vi "Magnetic Sweep 1.5.vi"() -> ()   [LabVIEW 2011]
uses:
  <vilib>/Math Plots/3D Math Plots/3D Contour/3D Contour XCtrl/3D Contour.xctl
  <vilib>/Math Plots/3D Math Plots/3D Contour/3D Contour Datatype/Public/Plot Helper (Vector).vi
  <vilib>/Math Plots/3D Math Plots/3D Contour/3D Contour Datatype/3D Contour Datatype.lvclass
panel:
  out "Heater":bool
  out "Persistent switch ready":bool
  out "error out 6":errorcluster
  in  "Temperature\nlower limite":dbl
  out "Ramping rate command":string
  out "Target field command":string
  out "error out 5":errorcluster
  in  "error out 4":errorcluster
  out "String":string="Persistent switch is not on"
  in  "Set parameter":bool
  out "status":string
  out "PID command":string
  out "setpoint command":string
  out "setpoint":dbl
  out "3D Contour \n(Ramp down)":refnum<class "3D Plot Datatype.lvclass">[](xcontrol)
  out "3D Contour\n(Ramp up)":refnum<class "3D Plot Datatype.lvclass">[](xcontrol)
  in  "stop":bool
  out "error out 3":errorcluster
  out "error out 2":errorcluster
  in  "Contour plot (ramp down)":path
  in  "Raw data (ramp down)":path
  out "Elapsed Time (s)":dbl
  out "Iteration":i32
  in  "error out":errorcluster
  out "Initial Temperature":string
  out "Zero field reached":bool
  out "Target field reached":bool
  in  "Temperature\nupper limite":dbl
  in  "Temperature\nramping step":dbl
  in  "Heater range":i16(ring) items=["High", "Medium", "Low"]
  in  "D gain":dbl
  in  "I gain":dbl
  in  "P gain":dbl
  in  "Contour plot (ramp up)":path
  out "Time elapsed":string
  in  "Timer":bool caption="Reset"
  in  "date format":enum16{"short", "long", "abbreviated"}(ring)
  in  "Save":bool
  in  "Raw data (ramp  up)":path
  out "Temperature vs Time":cluster{dbl[], dbl[]}(graph)
  out "current time":timestamp
  out "Magnetic\nField":cluster{dbl[], dbl[]}(graph)
  out "Current Resistance":string
  out "Current Temperature":string
  out "Current Field":string
  out "Status":string
  in  "Field Sweep":bool
  in  "Magnetic field\nRamp rate":dbl
  in  "Traget Field":dbl
  out "Init Response":string
  in  "error in (no error)":errorcluster
  in  "IP Address":string
  in  "Ramp":bool
  in  "Update":bool
  in  "Ramp to Zero":bool
  in  "P Switch":bool
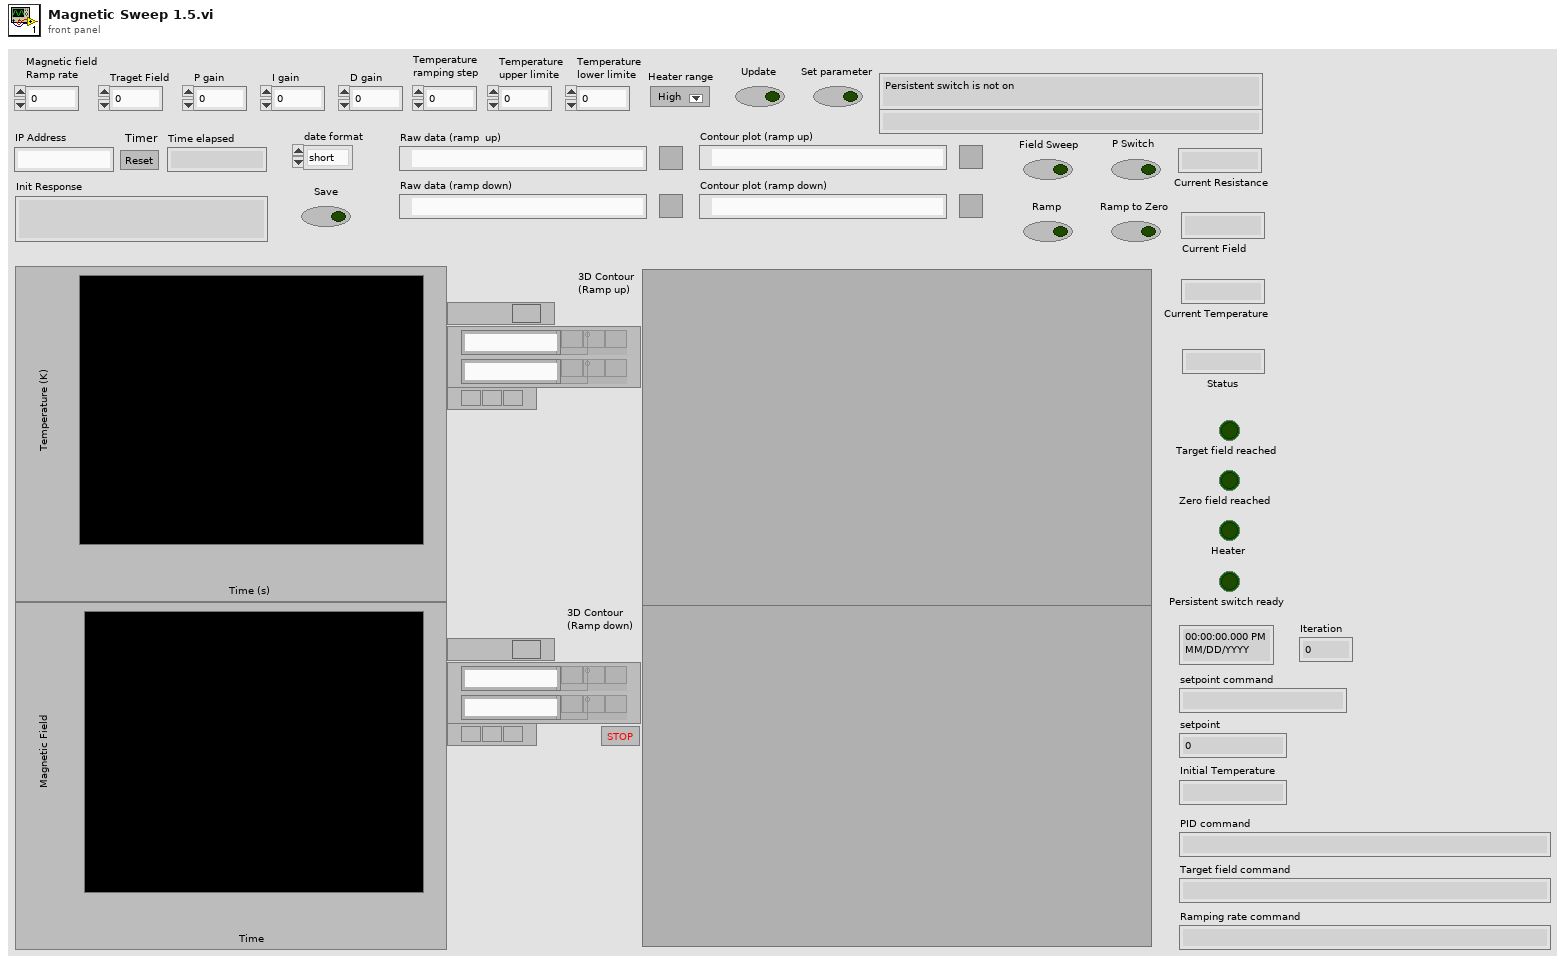
[diagram p1: front panel]
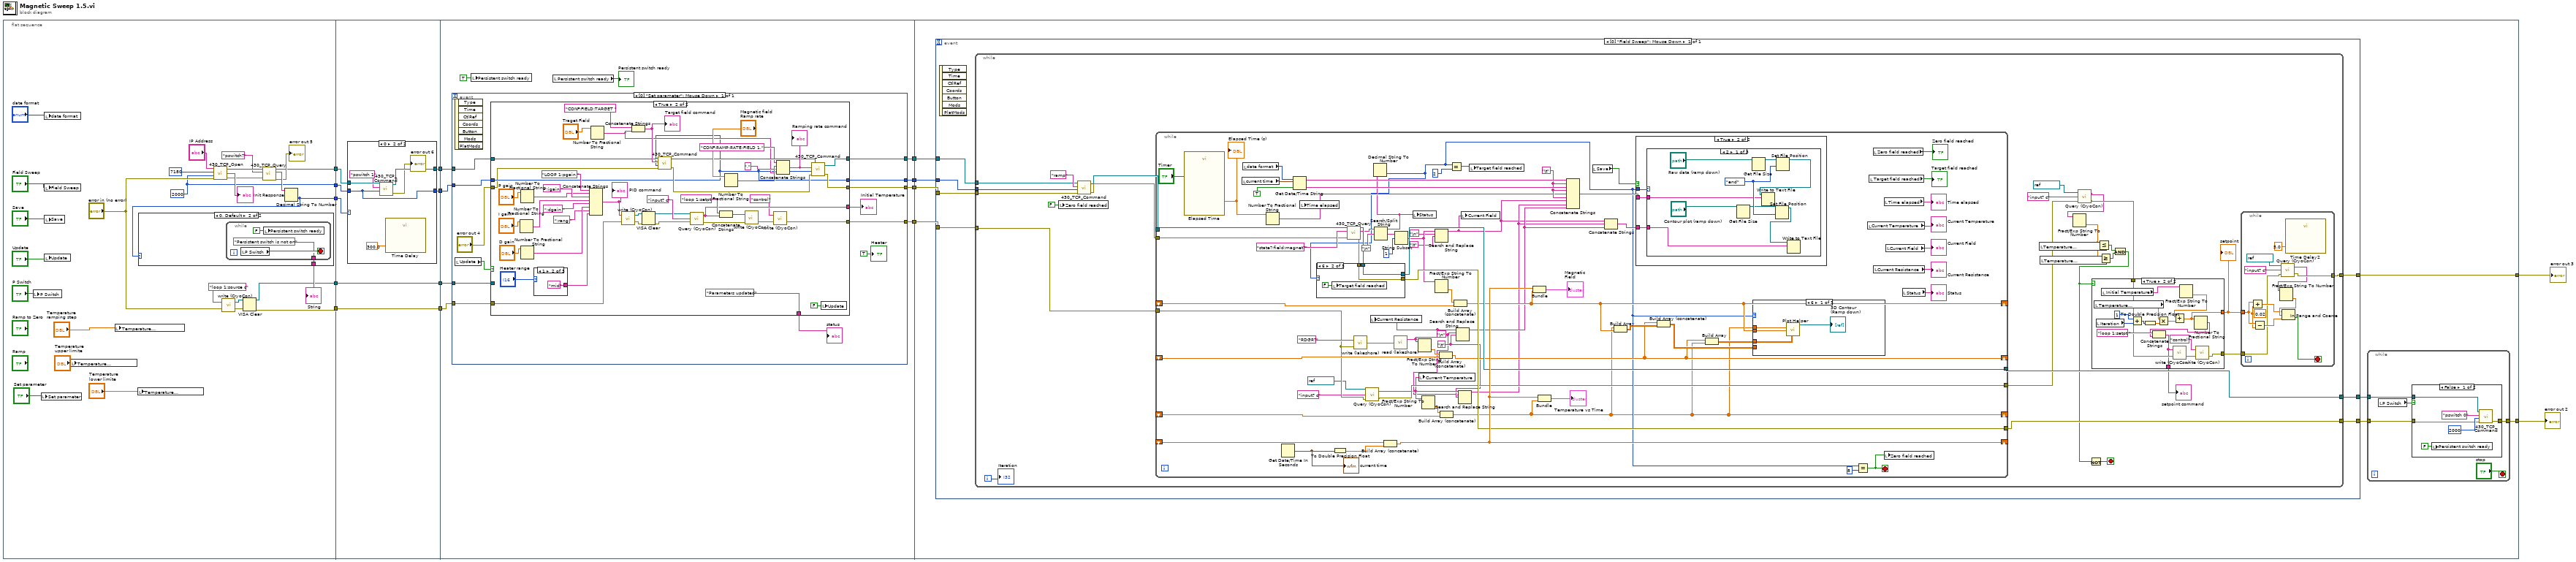
[diagram p0: block diagram]
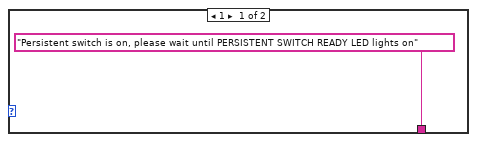
[diagram p2: hidden frame]
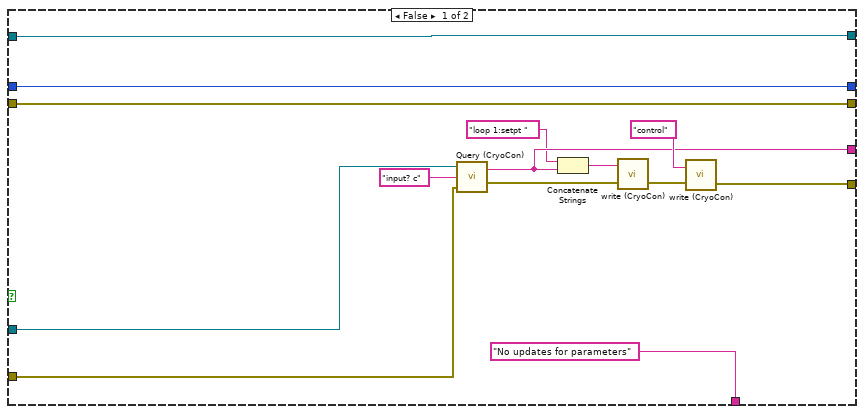
[diagram p4: hidden frame]
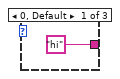
[diagram p5: hidden frame]
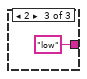
[diagram p6: hidden frame]
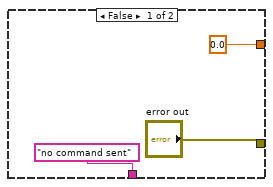
[diagram p8: hidden frame]
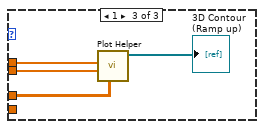
[diagram p10: hidden frame]
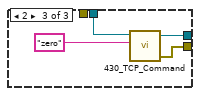
[diagram p12: hidden frame]
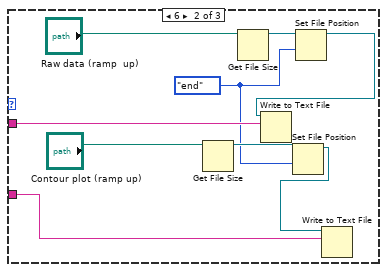
[diagram p14: hidden frame]
diagram:
  n1 = flat-sequence {
    tunnel: [w17] -> w9
    tunnel: [w20] -> w7
    tunnel: [w23] -> w5
    tunnel: [w21] -> w3
    tunnel: [w16] -> w1
    tunnel: w9 -> [w52]
    tunnel: [w50] -> w8
    tunnel: w7 -> [w51]
    tunnel: [w48] -> w6
    tunnel: w5 -> [w54]
    tunnel: [w54] -> w4
    tunnel: w3 -> [w53]
    tunnel: [w53] -> w2
    tunnel: w1 -> [w49]
    tunnel: w8 -> [w72]
    tunnel: w6 -> [w71]
    tunnel: w4 -> [w70]
    tunnel: [w69] -> w15
    tunnel: [w68] -> w12
    tunnel: [w67] -> w11
    tunnel: [w66] -> w10
    tunnel: w2 -> [w65]
    tunnel: w15 -> [w154]
    tunnel: [w153] -> w14
    tunnel: [w151] -> w13
    tunnel: w12 -> [w149]
    tunnel: w11 -> [w148]
    tunnel: w10 -> [w147]
    frame #0 {
      w20 = 2000 ("Timeout")
      n2 = local write "P Switch"("P Switch") -> ()
      n3 = local write "Set parameter"("Set parameter") -> ()
      n4 = local write "date format"("date format") -> ()
      n5 = local write "Field Sweep"("Field Sweep") -> ()
      n6 = local write "Save"("Save") -> ()
      n7 = local write "Update"("Update") -> ()
      n8 = local write "Temperature\nupper limite"("Temperature\nupper limite") -> ()
      n9 = local write "Temperature\nramping step"("Temperature\nramping step") -> ()
      n10 = local write "Temperature\nlower limite"("Temperature\nlower limite") -> ()
      n11 = call "430_TCP_Open.vi"("IP Address"="IP Address", "TCP Port"=7180, "timeout ms (2000)"=w20, "error in (no error)"="error in (no error)") -> ("connection ID"=w30:refnum<k5>, "Init Response"=→"Init Response":string, "error out"=w29:errorcluster)  [unwired: 2 in]
      n12 = call "write (CryoCon).vi"("error in (no error)"="error in (no error)", "write buffer"="loop 1:source c") -> ("error out"=w25:errorcluster, "VISA resource name out"=w24:refnum<visa-resource-name>)
      n13 = VISA Clear(VISA resource name=w24, error in (no error)=w25) -> (VISA resource name out=w21:refnum<visa-resource-name>, error out=w23:errorcluster)
      n14 = call "430_TCP_Query.vi"("error in (no error)"=w29, "Command"="pswitch?", "connection ID"=w30) -> ("error out"=→"error out 5":errorcluster, "Response"=w27:string, "connection ID out"=w17:refnum<k5>)  [unwired: 4 in, 2 out]
      n15 = Decimal String To Number(string=w27) -> (number=w16:i32)  [unwired: 2 in, 1 out]
      n16 = case shown="0, Default" w16 {
        tunnel: ["Persistent switch is on, please wait until PERSISTENT SWITCH READY LED lights on" w44] -> w22
        frame 1 {
        }
        frame 0, Default {
          n17 = while {
            tunnel: ["Persistent switch is not on"] -> w44
            stop <- w47 stop-if-true
            n18 = local read "P Switch"() -> (w47:bool)
            n19 = local write "Persistent switch ready"(FALSE ("Persistent switch ready")) -> ()
          }
        }
      }
      "String" <- w22
    }
    frame #1 {
      n20 = case shown="0" w49 {
        tunnel: w52 -> [w56 w62]
        tunnel: w51 -> [w55 w57]
        tunnel: [w56 w61] -> w50
        tunnel: [w55 w57] -> w48
        frame 1, Default {
        }
        frame 0 {
          n21 = call "430_TCP_Command.vi"("Timeout"=w57, "Command"="pswitch 1", "connection ID"=w62) -> ("error out"=→"error out 6":errorcluster, "connection ID out"=w61:refnum<k5>)  [unwired: 1 in, 1 out]
          n22 = call "Time Delay"("Delay Time (s)"=300.0) -> ()  [unwired: 10 in, 1 out]
        }
      }
    }
    frame #2 {
      n23 = event shown="[0] \"Set parameter\": Mouse Down" {
        selector: _ -> [_]
        dyn-events: _ -> [_]
        timeout: _ -> [_]
        tunnel: w72 -> [w85]
        tunnel: w71 -> [w84]
        tunnel: w70 -> [w83]
        tunnel: [w82] -> w69
        tunnel: [w81] -> w68
        tunnel: [w80] -> w67
        tunnel: [w79] -> w66
        tunnel: w65 -> [w75]
        event "Set parameter": Mouse Down {
          n24 = event-data() -> ()  [unwired: 1 in, 7 out]
          n25 = local read "Update"() -> (w76:bool)
          n26 = case shown="True" w76 {
            tunnel: w85 -> [w97 w141]
            tunnel: w84 -> [w98 w113]
            tunnel: w83 -> [w94 w120]
            tunnel: [w86 w101] -> w82
            tunnel: ["No updates for parameters" ("String") "Parameters updated" ("String")] -> w78
            tunnel: [w93 w115] -> w81
            tunnel: [w97 w114] -> w80
            tunnel: [w98 w113] -> w79
            tunnel: [w89 w105] -> w77
            tunnel: w75 -> [w95 _]
            tunnel: "error out 4" -> [w93 w100]
            frame False {
              n27 = call "Query (CryoCon).vi"("error in (no error)"=w94, "write buffer"="input? c", "VISA resource name 2"=w95) -> ("error out"=w87:errorcluster, "read buffer"=w89:string)
              n28 = Concatenate Strings("loop 1:setpt " ("write buffer"), w89) -> (w92:string)
              n29 = call "write (CryoCon).vi"("error in (no error)"=w87, "write buffer"=w92) -> ("error out"=w91:errorcluster)  [unwired: 1 out]
              n30 = call "write (CryoCon).vi"("error in (no error)"=w91, "write buffer"="control") -> ("error out"=w86:errorcluster)  [unwired: 1 out]
            }
            frame True {
              n31 = Number To Fractional String(number="I gain") -> (F-format string=w124:string)  [unwired: 3 in]
              n32 = Number To Fractional String(number="D gain") -> (F-format string=w122:string)  [unwired: 3 in]
              n33 = Number To Fractional String(number="P gain") -> (F-format string=w125:string)  [unwired: 3 in]
              n34 = case shown="1" "Heater range" {
                tunnel: ["hi" "mid" "low"] -> w117
                frame 0, Default {
                }
                frame 1 {
                }
                frame 2 {
                }
              }
              n35 = Concatenate Strings("LOOP 1:pgain " ("write buffer"), w125, ";igain " ("string"), w124, ";dgain " ("string"), w122, ";rang " ("string"), w117) -> (w121:string)
              "PID command" <- w121
              n36 = Number To Fractional String(number="Traget Field") -> (F-format string=w131:string)  [unwired: 3 in]
              n37 = call "write (CryoCon).vi"("error in (no error)"=w120, "write buffer"=w121) -> ("error out"=w112:errorcluster, "VISA resource name out"=w111:refnum<visa-resource-name>)
              n38 = Concatenate Strings("CONF:FIELD:TARGET ", w131) -> (w142:string)
              "Target field command" <- w142
              n39 = VISA Clear(VISA resource name=w111, error in (no error)=w112) -> (VISA resource name out=w108:refnum<visa-resource-name>, error out=w109:errorcluster)
              n40 = call "430_TCP_Command.vi"("error in (no error)"=w100, "Timeout"=w113, "Command"=w142, "connection ID"=w141) -> ("error out"=w140:errorcluster, "connection ID out"=w136:refnum<k5>)  [unwired: 1 out]
              n41 = call "Query (CryoCon).vi"("error in (no error)"=w109, "write buffer"="input? c", "VISA resource name 2"=w108) -> ("error out"=w107:errorcluster, "read buffer"=w105:string)
              n42 = Concatenate Strings("loop 1:setpt " ("write buffer"), w105) -> (w104:string)
              n43 = Number To Fractional String(number="Magnetic field\nRamp rate") -> (F-format string=w134:string)  [unwired: 3 in]
              n44 = call "write (CryoCon).vi"("error in (no error)"=w107, "write buffer"=w104) -> ("error out"=w103:errorcluster)  [unwired: 1 out]
              n45 = call "write (CryoCon).vi"("error in (no error)"=w103, "write buffer"="control") -> ("error out"=w101:errorcluster)  [unwired: 1 out]
              n46 = Concatenate Strings("CONF:RAMP:RATE:FIELD 1," ("string"), w134, "," ("string"), w131) -> (w137:string)
              "Ramping rate command" <- w137
              n47 = call "430_TCP_Command.vi"("error in (no error)"=w140, "Timeout"=w113, "Command"=w137, "connection ID"=w136) -> ("error out"=w115:errorcluster, "connection ID out"=w114:refnum<k5>)  [unwired: 1 out]
              n48 = local write "Update"(FALSE ("Update")) -> ()
            }
          }
          "Initial Temperature" <- w77
          "status" <- w78
          "Heater" <- TRUE ("Heater")
        }
      }
      n49 = local write "Persistent switch ready"(TRUE ("Persistent switch ready")) -> ()
      n50 = local read "Persistent switch ready"() -> (→"Persistent switch ready":bool)
    }
    frame #3 {
      n51 = event shown="[0] \"Field Sweep\": Mouse Down" {
        selector: _ -> [_]
        dyn-events: _ -> [_]
        timeout: _ -> [_]
        tunnel: w154 -> [w173]
        tunnel: [w172] -> w153
        tunnel: [w171] -> w152
        tunnel: [w170] -> w150
        tunnel: w149 -> [w169]
        tunnel: w148 -> [w168]
        tunnel: w147 -> [w167]
        event "Field Sweep": Mouse Down {
          n52 = event-data() -> ()  [unwired: 1 in, 7 out]
          n53 = while {
            tunnel: w173 -> [w198]
            tunnel: [w190] -> w172
            tunnel: [w189] -> w171
            tunnel: [w188] -> w170
            tunnel: w169 -> [w186]
            tunnel: w168 -> [w185]
            tunnel: w167 -> [w184]
            i -> [w195]
            stop <- w191 stop-if-true
            n54 = local write "Zero field reached"(FALSE ("Zero field reached")) -> ()
            n55 = call "430_TCP_Command.vi"("error in (no error)"=w186, "Timeout"=w184, "Command"="ramp", "connection ID"=w185) -> ("error out"=w200:errorcluster, "connection ID out"=w199:refnum<k5>)  [unwired: 1 out]
            n56 = while {
              shift-right: [w252] -> _
              shift-left: _ -> [w295]
              shift-right: [w232] -> _
              shift-left: _ -> [w300]
              shift-right: [w249] -> _
              shift-left: _ -> [w297]
              shift-right: [w290] -> _
              shift-left: _ -> [w291]
              tunnel: w200 -> [w280]
              tunnel: w199 -> [w279]
              tunnel: w198 -> [w246]
              tunnel: [w245] -> w182
              tunnel: [w260] -> w189
              tunnel: [w259] -> w188
              stop <- w263 stop-if-true
              w238 = "\t"
              w237 = "\n"
              w284 = "\t"
              n57 = call "Elapsed Time"("Reset"="Timer") -> ("Elapsed Time (s)"=w274:dbl)  [unwired: 11 in, 7 out]
              "Elapsed Time (s)" <- w274
              n58 = local read "current time"() -> (w282:timestamp)
              n59 = local read "date format"() -> (w276:enum16{"short", "long", "abbreviated"})
              n60 = Number To Fractional String(number=w274) -> (F-format string=w277:string)  [unwired: 3 in]
              n61 = Get Date/Time In Seconds() -> (seconds since 1Jan1904=w273:timestamp)
              "current time" <- w273
              n62 = Get Date/Time String(date format (0)=w276, seconds (now)=w282, want seconds? (F)=TRUE) -> (date string=w286:string, time string=w285:string)
              n63 = local write "Time elapsed"(w277) -> ()
              n64 = To Double Precision Float(number=w273) -> (double precision float=w292:dbl)
              n65 = call "430_TCP_Query.vi"("error in (no error)"=w280, "Command"="state?;field:magnet?", "connection ID"=w279) -> ("error out"=w247:errorcluster, "Response"=w258:string, "connection ID out"=w262:refnum<k5>)  [unwired: 4 in, 2 out]
              n66 = call "write (lakeshore).vi"("error in (no error)"=w246, "write buffer"="RDGR?") -> ("error out"=w299:errorcluster)
              n67 = call "Query (CryoCon).vi"("error in (no error)"=w246, "write buffer"="input? c", "VISA resource name 2"=refnum<visa-resource-name> "COM3") -> ("error out"=w245:errorcluster, "read buffer"=w240:string)
              n68 = Search/Split String(string=w258, search string/char (-)="\n") -> (substring before match=w257:string, match + rest of string=w256:string)  [unwired: 1 in, 1 out]
              n69 = Decimal String To Number(string=w257) -> (number=w248:i32)  [unwired: 2 in, 1 out]
              n70 = case shown="6" w248 {
                tunnel: [w310 w312 w317] -> w259
                tunnel: w262 -> [w311 w314 w316]
                tunnel: [w311 w314 w315] -> w260
                tunnel: w247 -> [w310 w312 _]
                frame 0, Default {
                }
                frame 6 {
                  n71 = local write "Target field reached"(FALSE ("Target field reached")) -> ()
                }
                frame 2 {
                  n72 = call "430_TCP_Command.vi"("Command"="zero", "connection ID"=w316) -> ("error out"=w317:errorcluster, "connection ID out"=w315:refnum<k5>)  [unwired: 2 in, 1 out]
                }
              }
              n73 = Build Array (concatenate)(w291, w292) -> (w290:dbl[])
              n74 = call "read (lakeshore).vi"("error in (no error)"=w299) -> ("read buffer"=w242:string)  [unwired: 1 out]
              n75 = local write "Current Resistance"(w242) -> ()
              n76 = String Subset(string=w256, offset (0)=1) -> (substring=w235:string)  [unwired: 1 in]
              n77 = local write "Status"(w257) -> ()
              n78 = Fract/Exp String To Number(string=w242) -> (number=w293:dbl)  [unwired: 3 in, 1 out]
              n79 = local write "Current Temperature"(w240) -> ()
              n80 = Fract/Exp String To Number(string=w240) -> (number=w294:dbl)  [unwired: 3 in, 1 out]
              n81 = Search and Replace String(input string=w235, search string="\n", replace string="\t") -> (result string=w236:string)  [unwired: 5 in, 3 out]
              n82 = Fract/Exp String To Number(string=w235) -> (number=w296:dbl)  [unwired: 3 in, 1 out]
              n83 = Build Array (concatenate)(w293, w297) -> (w249:dbl[])
              n84 = Build Array (concatenate)(w294, w300) -> (w232:dbl[])
              n85 = Equal?(x=w248, y=2) -> (x = y?=w278:bool)
              n86 = Build Array (concatenate)(w296, w295) -> (w252:dbl[])
              n87 = Search and Replace String(input string=w242, search string=w237, replace string=w238) -> (result string=w241:string)  [unwired: 5 in, 3 out]
              n88 = Search and Replace String(input string=w240, search string=w237, replace string=w238) -> (result string=w239:string)  [unwired: 5 in, 3 out]
              n89 = local write "Current Field"(w236) -> ()
              n90 = local write "Target field reached"(w278) -> ()
              n91 = Bundle(w290, w252) -> (→"Magnetic\nField":cluster{dbl[], dbl[]})  [unwired: 1 in]
              n92 = Bundle(w290, w232) -> (→"Temperature vs Time":cluster{dbl[], dbl[]})  [unwired: 1 in]
              n93 = Concatenate Strings(w286, w284, w285, w284, w277, w284, w236, w239, w241) -> (w289:string)
              n94 = local read "Save"() -> (w272:bool)
              n95 = Concatenate Strings(w236, w239, w241) -> (w283:string)
              n96 = Build Array(w232, w252) -> (w261:dbl[][])
              n97 = case shown="True" w272 {
                tunnel: w289 -> [_ w321]
                tunnel: w283 -> [_ w320]
                tunnel: w248 -> [_ w319]
                frame False {
                }
                frame True {
                  n98 = case shown="2" w319 {
                    tunnel: w321 -> [w323 w339 _]
                    tunnel: w320 -> [w322 w333 _]
                    frame 2 {
                      w329 = enum16{"start", "end", "current"}."end" ("from (0:start)")
                      n99 = Get File Size(file="Contour plot (ramp down)") -> (refnum out=w328:refnum<file>)  [unwired: 1 in, 2 out]
                      n100 = Get File Size(file="Raw data (ramp down)") -> (refnum out=w325:refnum<file>)  [unwired: 1 in, 2 out]
                      n101 = Set File Position(refnum=w328, from (0:start)=w329) -> (refnum out=w330:refnum<file>)  [unwired: 2 in, 1 out]
                      n102 = Set File Position(refnum=w325, from (0:start)=w329) -> (refnum out=w326:refnum<file>)  [unwired: 2 in, 1 out]
                      n103 = Write to Text File(file (use dialog)=w326, text=w323) -> ()  [unwired: 2 in, 3 out]
                      n104 = Write to Text File(file (use dialog)=w330, text=w322) -> ()  [unwired: 2 in, 3 out]
                    }
                    frame 6 {
                      w332 = enum16{"start", "end", "current"}."end" ("from (0:start)")
                      n105 = Get File Size(file="Contour plot (ramp up)") -> (refnum out=w334:refnum<file>)  [unwired: 1 in, 2 out]
                      n106 = Get File Size(file="Raw data (ramp  up)") -> (refnum out=w337:refnum<file>)  [unwired: 1 in, 2 out]
                      n107 = Set File Position(refnum=w334, from (0:start)=w332) -> (refnum out=w331:refnum<file>)  [unwired: 2 in, 1 out]
                      n108 = Set File Position(refnum=w337, from (0:start)=w332) -> (refnum out=w336:refnum<file>)  [unwired: 2 in, 1 out]
                      n109 = Write to Text File(file (use dialog)=w336, text=w339) -> ()  [unwired: 2 in, 3 out]
                      n110 = Write to Text File(file (use dialog)=w331, text=w333) -> ()  [unwired: 2 in, 3 out]
                    }
                    frame Default {
                    }
                  }
                }
              }
              n111 = Build Array (concatenate)(w249, w261) -> (w250:dbl[][])
              n112 = Build Array(w249, w232) -> (w251:dbl[][])
              n113 = case shown="6" w248 {
                tunnel: w232 -> [w304 _ w308]
                tunnel: w252 -> [w303 _ w307]
                tunnel: w251 -> [w302 _ w306]
                tunnel: w250 -> [_ _ _]
                frame 6 {
                  n114 = call-poly <vilib>:"Plot Helper.vi"("z matrix"=w302, "y vector"=w303, "x vector"=w304) -> ("3D Plot lvclass Array out"=→"3D Contour \n(Ramp down)":refnum<class "3D Plot Datatype.lvclass">[])  [unwired: 3 in, 5 out]
                }
                frame 0, Default {
                }
                frame 1 {
                  n115 = call-poly <vilib>:"Plot Helper.vi"("z matrix"=w306, "y vector"=w307, "x vector"=w308) -> ("3D Plot lvclass Array out"=→"3D Contour\n(Ramp up)":refnum<class "3D Plot Datatype.lvclass">[])  [unwired: 3 in, 5 out]
                }
              }
              n116 = Equal?(x=w248, y=8) -> (x = y?=w263:bool)
              n117 = local read "Current Temperature"() -> (→"Current Temperature":string)
              n118 = local read "Target field reached"() -> (→"Target field reached":bool)
              n119 = local read "Zero field reached"() -> (→"Zero field reached":bool)
              n120 = local read "Current Resistance"() -> (→"Current Resistance":string)
              n121 = local read "Time elapsed"() -> (→"Time elapsed":string)
              n122 = local write "Zero field reached"(w263) -> ()
              n123 = local read "Current Field"() -> (→"Current Field":string)
              n124 = local read "Status"() -> (→"Status":string)
            }
            n125 = local read "Temperature\nupper limite"() -> (w192:dbl)
            n126 = local read "Temperature\nlower limite"() -> (w177:dbl)
            n127 = call "Query (CryoCon).vi"("error in (no error)"=w182, "write buffer"="input? c", "VISA resource name 2"=refnum<visa-resource-name> "COM3") -> ("error out"=w181:errorcluster, "read buffer"=w180:string)
            n128 = Fract/Exp String To Number(string=w180) -> (number=w178:dbl)  [unwired: 3 in, 1 out]
            n129 = Less Or Equal?(x=w178, y=w192) -> (x <= y?=w175:bool)
            n130 = Greater Or Equal?(x=w178, y=w177) -> (x >= y?=w176:bool)
            n131 = And(x=w175, y=w176) -> (x .and. y?=w174:bool)
            n132 = Not(x=w174) -> (.not. x?=w191:bool)
            n133 = case shown="True" w174 {
              tunnel: w181 -> [_ w229]
              tunnel: ["error out" w218] -> w197
              tunnel: [0.0 w226] -> w196
              tunnel: ["no command sent" w222] -> w187
              frame False {
              }
              frame True {
                n134 = local read "Temperature\nramping step"() -> (w224:dbl)
                n135 = local read "Iteration"() -> (w221:i32)
                n136 = local read "Initial Temperature"() -> (w228:string)
                n137 = Add(x=1, y=w221) -> (x+y=w220:i32)
                n138 = To Double Precision Float(number=w220) -> (double precision float=w223:dbl)
                n139 = Multiply(x=w224, y=w223) -> (x*y=w225:dbl)
                n140 = Fract/Exp String To Number(string=w228) -> (number=w227:dbl)  [unwired: 3 in, 1 out]
                n141 = Add(x=w227, y=w225) -> (x+y=w226:dbl)
                n142 = Number To Fractional String(number=w226) -> (F-format string=w230:string)  [unwired: 3 in]
                n143 = Concatenate Strings("loop 1:setpt " ("write buffer"), w230) -> (w222:string)
                n144 = call "write (CryoCon).vi"("error in (no error)"=w229, "write buffer"=w222) -> ("error out"=w217:errorcluster)  [unwired: 1 out]
                n145 = call "write (CryoCon).vi"("error in (no error)"=w217, "write buffer"="control") -> ("error out"=w218:errorcluster)  [unwired: 1 out]
              }
            }
            "setpoint" <- w196
            "setpoint command" <- w187
            n146 = while {
              tunnel: w197 -> [w204]
              tunnel: w196 -> [w211]
              tunnel: [w203] -> w190
              stop <- w207 stop-if-true
              w208 = 0.02 ("y")
              n147 = Add(x=w211, y=w208) -> (x+y=w210:dbl)
              n148 = Subtract(x=w211, y=w208) -> (x-y=w209:dbl)
              n149 = call "Query (CryoCon).vi"("error in (no error)"=w204, "write buffer"="input? c", "VISA resource name 2"=refnum<visa-resource-name> "COM3") -> ("error out"=w203:errorcluster, "read buffer"=w202:string)
              n150 = Fract/Exp String To Number(string=w202) -> (number=w212:dbl)  [unwired: 3 in, 1 out]
              n151 = In Range and Coerce(upper limit=w210, x=w212, lower limit=w209) -> (In Range?=w207:bool)  [unwired: 1 out]
              n152 = call "Time Delay2"("Delay Time (s)"=5.0) -> ()  [unwired: 10 in, 1 out]
            }
            "Iteration" <- w195
          }
        }
      }
      n153 = while {
        tunnel: w152 -> [w159]
        tunnel: [w157] -> w151
        tunnel: w150 -> [w156]
        stop <- "stop" stop-if-true
        n154 = local read "P Switch"() -> (w158:bool)
        n155 = case shown="False" w158 {
          tunnel: w159 -> [w164 _]
          tunnel: [w162 w166] -> w157
          tunnel: w156 -> [w161 w166]
          frame False {
            n156 = local write "Persistent switch ready"(FALSE ("Persistent switch ready")) -> ()
            n157 = call "430_TCP_Command.vi"("error in (no error)"=w161, "Timeout"=2000, "Command"="pswitch 0", "connection ID"=w164) -> ("error out"=w162:errorcluster)  [unwired: 2 out]
          }
          frame True {
          }
        }
      }
    }
  }
  "error out 2" <- w13
  "error out 3" <- w14
